vi "Numeric_bins.vi"(0 "Values":dbl[](array[numeric]) format="%.4f", 1 "Tolerance":dbl=0.02 format="%.3f") -> (2 "Bin Centres":dbl[](array[numeric]) format="%.4f", 3 "No of points in bins":i32[](array[numeric]), 4 "Bin Index":i32[](array[numeric]))   [LabVIEW 2015]
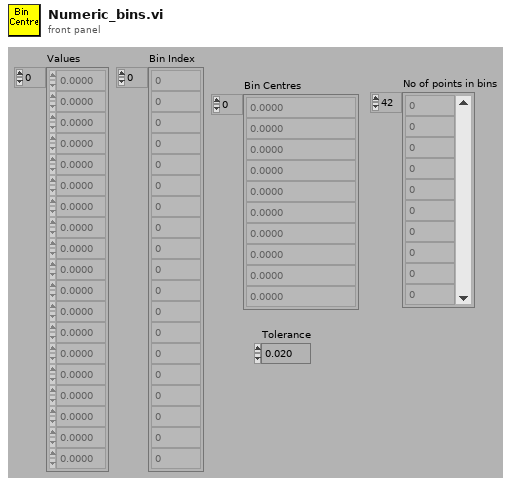
[diagram p1: front panel]
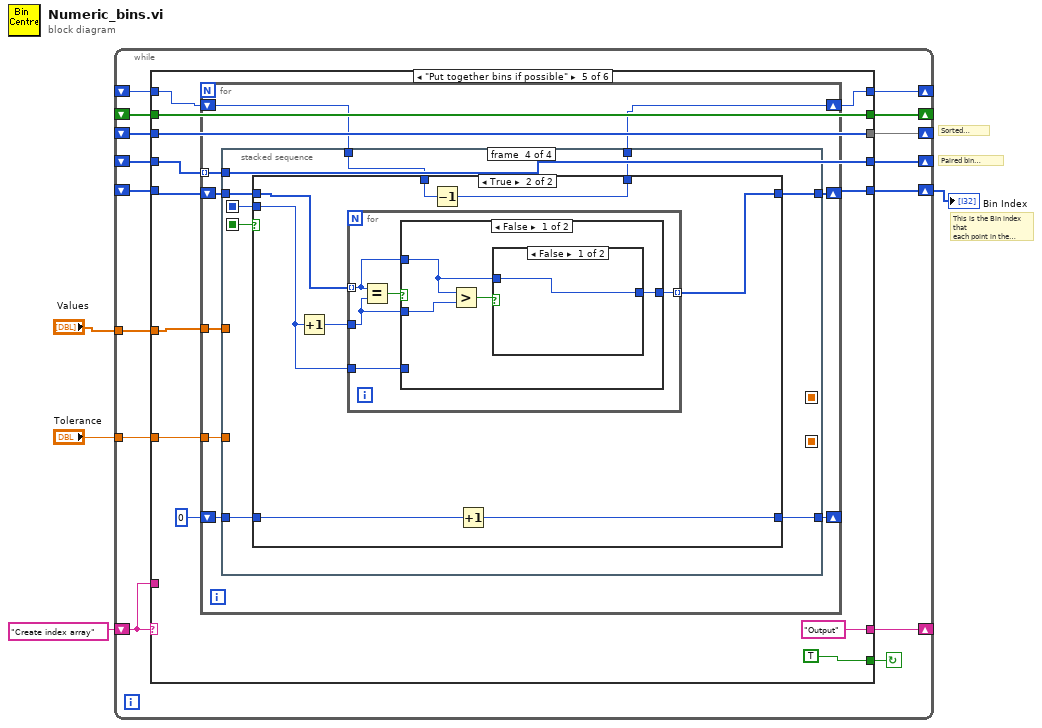
[diagram p0: block diagram]
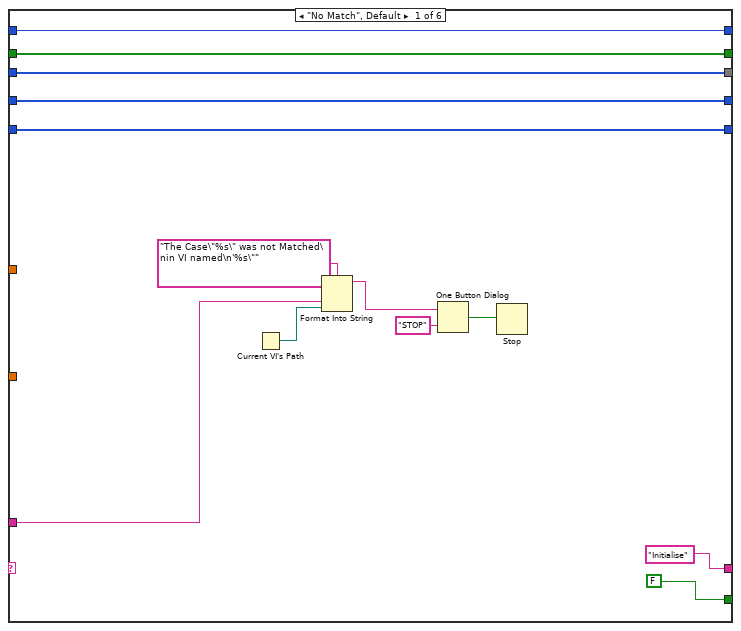
[diagram p2: hidden frame]
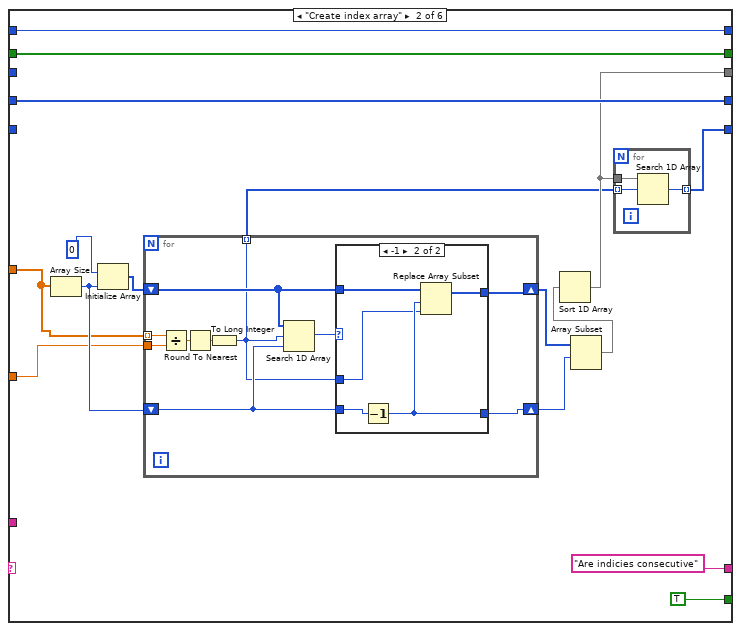
[diagram p3: hidden frame]
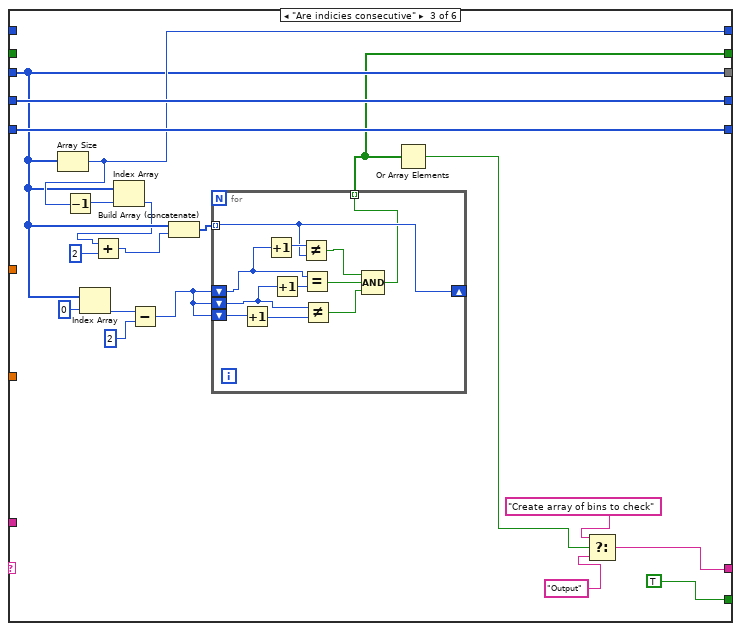
[diagram p5: hidden frame]
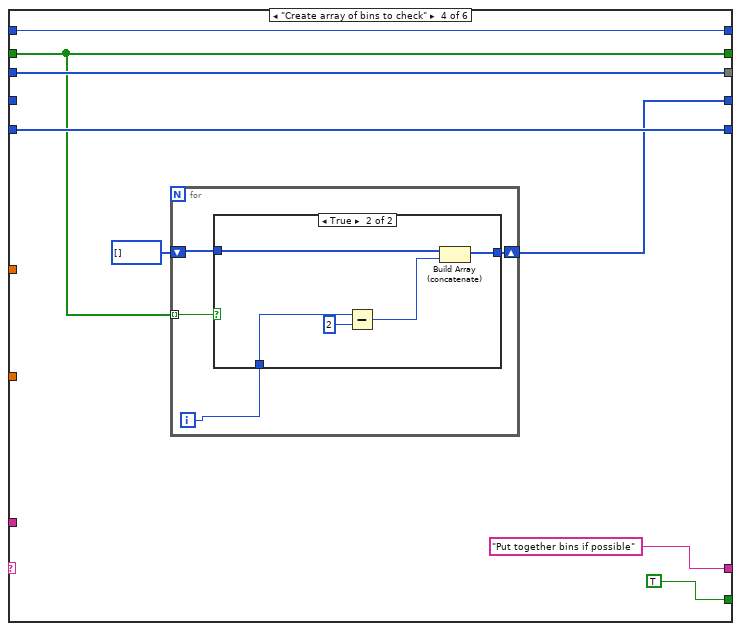
[diagram p6: hidden frame]
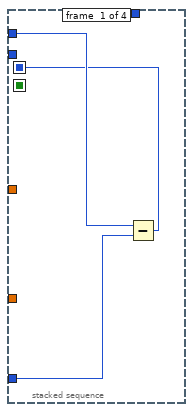
[diagram p8: hidden frame]
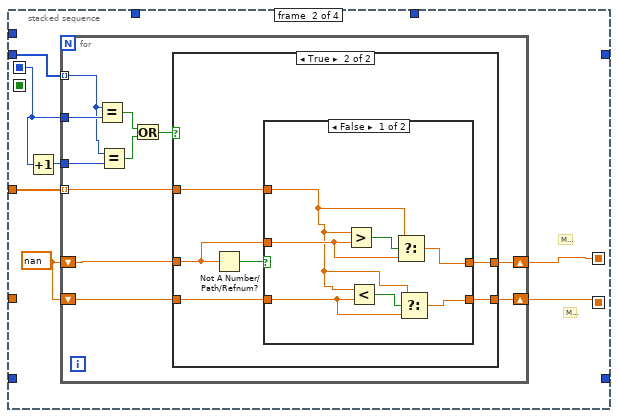
[diagram p9: hidden frame]
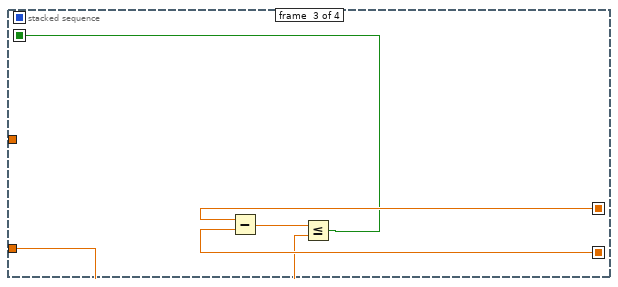
[diagram p12: hidden frame]
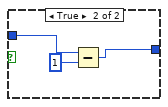
[diagram p14: hidden frame]
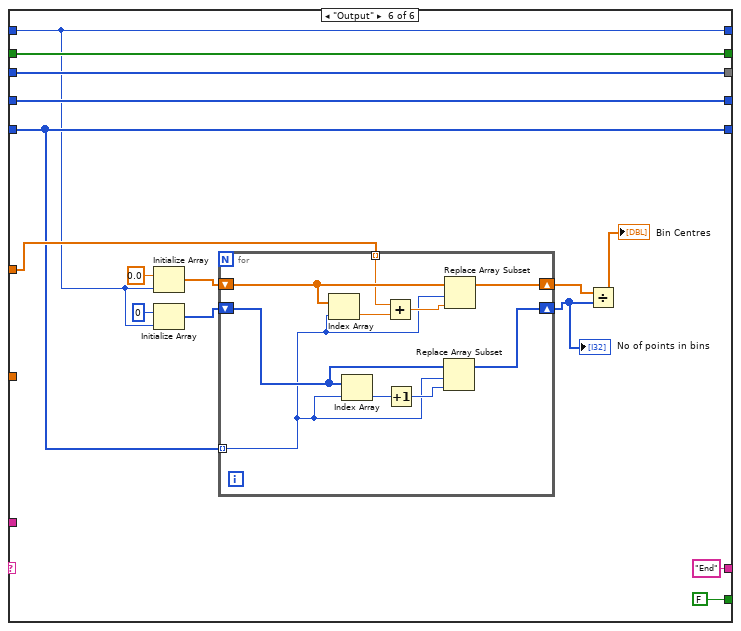
[diagram p16: hidden frame]
diagram:
  # "Paired bin numbers"
  # "This is the Bin index that\neach point in the values\narray falls into"
  # "Sorted indicies"
  n1 = while {
    shift-left: "Create index array" -> [w17]
    shift-right: [w18] -> _
    shift-right: [w16] -> _
    shift-left: _ -> [w11]
    shift-right: [w15] -> _
    shift-left: _ -> [w12]
    tunnel: "Values" -> [w14]
    tunnel: "Tolerance" -> [w13]
    shift-right: [w10] -> _
    shift-left: _ -> [w8]
    shift-right: [w9] -> w1
    shift-left: _ -> [w7]
    shift-right: [w6] -> _
    shift-left: _ -> [w5]
    stop <- w19 continue-if-true
    n2 = case shown="\"Put together bins if possible\"" w17 {
      tunnel: [FALSE TRUE TRUE TRUE TRUE FALSE] -> w19
      tunnel: ["Initialise" "Are indicies consecutive" w81 "Put together bins if possible" "Output" "End"] -> w18
      tunnel: w17 -> [w27 _ _ _ _ _]
      tunnel: [w23 w45 w75 w104 w127 w220] -> w16
      tunnel: [w24 w43 w70 w102 w126 w221] -> w15
      tunnel: w14 -> [_ w38 _ _ w124 w222]
      tunnel: w13 -> [_ w37 _ _ w123 _]
      tunnel: w12 -> [w24 w43 _ w102 w126 w221]
      tunnel: w11 -> [w23 _ w75 w104 w127 w220]
      tunnel: [w22 w46 w86 w99 w125 w215] -> w10
      tunnel: [w21 w44 w85 w105 w121 w217] -> w9
      tunnel: w8 -> [w22 w46 w86 _ w125 w215]
      tunnel: w7 -> [w21 _ w85 w105 w122 w217]
      tunnel: [w20 w42 w77 w101 w119 w214] -> w6
      tunnel: w5 -> [w20 w42 _ w101 w118 w214]
      frame "No Match", Default {
        n3 = Current VI's Path() -> (path=w26:path)
        n4 = Format Into String(format string="The Case\"%s\" was not Matched\nin VI named\n'%s\"" ("Format String"), w27, w26) -> (resulting string=w30:string)  [unwired: 2 in, 1 out]
        n5 = One Button Dialog(message=w30, button name ("OK")="STOP") -> (true=w28:bool)
        n6 = Stop(stop? (T)=w28) -> ()
      }
      frame "Create index array" {
        n7 = Array Size(array=w38) -> (size(s)=w39:i32)
        n8 = Initialize Array(0, w39) -> (w40:i32[])
        n9 = for {
          shift-right: [w60] -> w35
          shift-left: w40 -> [w59]
          shift-right: [w53] -> w36
          shift-left: w39 -> [w54]
          tunnel: w38 -> [w57] mode=indexing
          tunnel: w37 -> [w56]
          tunnel: [w52] -> w33 mode=indexing
          n10 = Divide(x=w57, y=w56) -> (x/y=w55:dbl)
          n11 = Round To Nearest(number=w55) -> (nearest integer value=w58:dbl)
          n12 = To Long Integer(number=w58) -> (32bit integer=w52:i32)
          n13 = Search 1D Array(1D array=w59, element=w52, start index (0)=w54) -> (index of element=w61:i32)
          n14 = case shown="-1" w61 {
            tunnel: w59 -> [w63 w68]
            tunnel: w52 -> [_ w64]
            tunnel: [w63 w67] -> w60
            tunnel: w54 -> [w62 w66]
            tunnel: [w62 w65] -> w53
            frame 0, Default {
            }
            frame -1 {
              n15 = Decrement(x=w66) -> (x-1=w65:i32)
              n16 = Replace Array Subset(array=w68, new element=w64, index=w65) -> (w67:i32[])
            }
          }
        }
        n17 = Array Subset(array=w35, index=w36) -> (w34:i32[])  [unwired: 1 in]
        n18 = Sort 1D Array(array=w34) -> (sorted array=w45:i32[])
        n19 = for {
          tunnel: w45 -> [w51]
          tunnel: w33 -> [w50] mode=indexing
          tunnel: [w49] -> w44 mode=indexing
          n20 = Search 1D Array(1D array=w51, element=w50) -> (index of element=w49:i32)  [unwired: 1 out]
        }
      }
      frame "Are indicies consecutive" {
        n21 = Array Size(array=w75) -> (size(s)=w77:i32)
        n22 = Decrement(x=w77) -> (x-1=w76:i32)
        n23 = Index Array(array=w75, index=0) -> (element=w83:i32)
        n24 = Index Array(array=w75, index=w76) -> (element=w74:i32)
        n25 = Add(x=w74, y=2) -> (x+y=w72:i32)
        n26 = Subtract(x=w83, y=2) -> (x-y=w78:i32)
        n27 = Build Array (concatenate)(w75, w72) -> (w71:i32[])
        n28 = for {
          shift-right: [w92] -> _
          shift-left: w78 -> [w94]
          tunnel: w71 -> [w92] mode=indexing
          tunnel: [w88] -> w70 mode=indexing
          shift-left: w78 -> [w96]
          shift-left: w78 -> [w98]
          n29 = Increment(x=w98) -> (x+1=w97:i32)
          n30 = Increment(x=w94) -> (x+1=w93:i32)
          n31 = Increment(x=w96) -> (x+1=w95:i32)
          n32 = Not Equal?(x=w93, y=w92) -> (x != y?=w91:bool)
          n33 = Equal?(x=w94, y=w95) -> (x = y?=w90:bool)
          n34 = Not Equal?(x=w96, y=w97) -> (x != y?=w89:bool)
          n35 = Compound Arithmetic op=AND(w91, w90, w89) -> (w88:bool)
        }
        n36 = Or Array Elements(Boolean array=w70) -> (logical OR=w69:bool)
        n37 = Select(t="Create array of bins to check", s=w69, f="Output") -> (s? t:f=w81:string)
      }
      frame "Create array of bins to check" {
        n38 = for {
          tunnel: w102 -> [w110] mode=indexing
          shift-right: [w107] -> w99
          shift-left: i32[] [] -> [w108]
          i -> [w109]
          n39 = case shown="True" w110 {
            tunnel: w109 -> [_ w116]
            tunnel: w108 -> [w111 w114]
            tunnel: [w111 w112] -> w107
            frame False {
            }
            frame True {
              n40 = Subtract(x=w116, y=2) -> (x-y=w113:i32)
              n41 = Build Array (concatenate)(w114, w113) -> (w112:i32[])
            }
          }
        }
      }
      frame "Put together bins if possible" {
        n42 = for {
          tunnel: w125 -> [w137] mode=indexing
          tunnel: w124 -> [w136]
          tunnel: w123 -> [w135]
          shift-right: [w134] -> w121
          shift-left: w122 -> [w133]
          shift-right: [w131] -> w119
          shift-left: w118 -> [w132]
          shift-right: [w130] -> _
          shift-left: 0 -> [w129]
          n43 = stacked-sequence {
            seq-local: [_ w145 _ _] -> [_ _ w179 _]
            seq-local: [_ w144 _ _] -> [_ _ w178 _]
            seq-local: [_ _ w175 _] -> [_ _ _ w187]
            seq-local: [w138 _ _ _] -> [_ w141 _ w180]
            tunnel: w137 -> [w140 _ _ _]
            tunnel: w136 -> [_ w146 _ _]
            tunnel: w135 -> [_ _ w176 _]
            tunnel: [_ _ _ w186] -> w134
            tunnel: w133 -> [_ w142 _ w185]
            tunnel: w132 -> [_ _ _ w184]
            tunnel: [_ _ _ w183] -> w131
            tunnel: [_ _ _ w182] -> w130
            tunnel: w129 -> [w139 _ _ w181]
            frame #0 {
              n44 = Subtract(x=w140, y=w139) -> (x-y=w138:i32)
            }
            frame #1 {
              w147 = nan
              # "Min"
              # "Max"
              n45 = Increment(x=w141) -> (x+1=w143:i32)
              n46 = for {
                tunnel: w141 -> [w158]
                shift-right: [w152] -> w145
                shift-left: w147 -> [w154]
                shift-right: [w151] -> w144
                shift-left: w147 -> [w150]
                tunnel: w146 -> [w153] mode=indexing
                tunnel: w143 -> [w149]
                tunnel: w142 -> [w148] mode=indexing
                n47 = Equal?(x=w148, y=w158) -> (x = y?=w156:bool)
                n48 = Equal?(x=w148, y=w149) -> (x = y?=w157:bool)
                n49 = Or(x=w156, y=w157) -> (x .or. y?=w155:bool)
                n50 = case shown="True" w155 {
                  tunnel: w154 -> [w160 w162]
                  tunnel: w153 -> [_ w165]
                  tunnel: [w160 w164] -> w152
                  tunnel: [w159 w163] -> w151
                  tunnel: w150 -> [w159 w161]
                  frame False {
                  }
                  frame True {
                    n51 = Not A Number/Path/Refnum?(number/path/refnum=w162) -> (NaN/Path/Refnum?=w166:bool)
                    n52 = case shown="False" w166 {
                      tunnel: w165 -> [w169 w174]
                      tunnel: [w171 w174] -> w164
                      tunnel: [w167 w174] -> w163
                      tunnel: w162 -> [w172 _]
                      tunnel: w161 -> [w168 _]
                      frame False {
                        n53 = Greater?(x=w169, y=w172) -> (0:w173:bool)
                        n54 = Less?(x=w169, y=w168) -> (x < y?=w170:bool)
                        n55 = Select(t=w169, s=w173, f=w172) -> (s? t:f=w171:dbl)
                        n56 = Select(t=w169, s=w170, f=w168) -> (s? t:f=w167:dbl)
                      }
                      frame True {
                      }
                    }
                  }
                }
              }
            }
            frame #2 {
              n57 = Subtract(x=w179, y=w178) -> (x-y=w177:dbl)
              n58 = Less Or Equal?(x=w177, y=w176) -> (x <= y?=w175:bool)
            }
            frame #3 {
              n59 = case shown="True" w187 {
                tunnel: [w190 w196] -> w186
                tunnel: w185 -> [w190 w197]
                tunnel: w184 -> [w189 w195]
                tunnel: [w189 w194] -> w183
                tunnel: [w188 w191] -> w182
                tunnel: w181 -> [w188 w192]
                tunnel: w180 -> [_ w193]
                frame False {
                }
                frame True {
                  n60 = Increment(x=w193) -> (x+1=w198:i32)
                  n61 = for {
                    tunnel: w198 -> [w199]
                    tunnel: w197 -> [w200] mode=indexing
                    tunnel: [w202] -> w196 mode=indexing
                    tunnel: w193 -> [w201]
                    n62 = Equal?(x=w200, y=w199) -> (x = y?=w203:bool)
                    n63 = case shown="False" w203 {
                      tunnel: [w204 w212] -> w202
                      tunnel: w201 -> [_ w212]
                      tunnel: w200 -> [w205 _]
                      tunnel: w199 -> [w207 _]
                      frame False {
                        n64 = Greater?(x=w205, y=w207) -> (0:w206:bool)
                        n65 = case shown="False" w206 {
                          tunnel: w205 -> [w208 w211]
                          tunnel: [w208 w209] -> w204
                          frame False {
                          }
                          frame True {
                            n66 = Subtract(x=w211, y=1) -> (x-y=w209:i32)
                          }
                        }
                      }
                      frame True {
                      }
                    }
                  }
                  n67 = Decrement(x=w195) -> (x-1=w194:i32)
                  n68 = Increment(x=w192) -> (x+1=w191:i32)
                }
              }
            }
          }
        }
      }
      frame "Output" {
        n69 = Initialize Array(0.0 ("element"), w214) -> (w224:dbl[])
        n70 = Initialize Array(0 ("element"), w214) -> (w226:i32[])
        n71 = for {
          shift-right: [w236] -> w227
          shift-left: w224 -> [w237]
          shift-right: [w235] -> w213
          shift-left: w226 -> [w234]
          tunnel: w222 -> [w229] mode=indexing
          tunnel: w217 -> [w228] mode=indexing
          n72 = Index Array(array=w237, index=w228) -> (element=w231:dbl)
          n73 = Index Array(array=w234, index=w228) -> (element=w233:i32)
          n74 = Add(x=w229, y=w231) -> (x+y=w230:dbl)
          n75 = Increment(x=w233) -> (x+1=w232:i32)
          n76 = Replace Array Subset(array=w234, new element=w232, index=w228) -> (w235:i32[])
          n77 = Replace Array Subset(array=w237, new element=w230, index=w228) -> (w236:dbl[])
        }
        "No of points in bins" <- w213
        n78 = Divide(x=w227, y=w213) -> (x/y=→"Bin Centres":dbl[])
      }
    }
  }
  "Bin Index" <- w1
